vi "SQLite Count Template.vi"(6 "Range":T1, 7 "Filter":cluster{}, 8 "Error in":errorcluster, 10 "Filter Fields":string[](array[combo]), 11 "SQLite Connection in":refnum<class "Connection.lvclass">) -> (0 "Error out":errorcluster, 2 "Count":i32, 3 "SQLite Connection out":refnum<class "Connection.lvclass">)   [LabVIEW 2021]
uses:
  <vilib>/drjdpowell/SQLite Library/SQL Statement/SQL Statement.lvclass
  <vilib>/drjdpowell/SQLite Library/SQL Connection/Connection.lvclass
  edt.lib/sqlite.lib/EDT SQLite+.lvlib
  edt.lib/sqlite.lib/SQLite Range.ctl
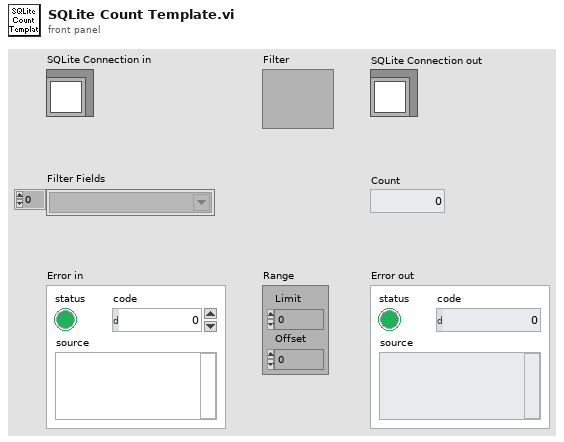
[diagram p1: front panel]
types:
  T1 = typedef "EDT SQLite+.lvlib/SQLite Range.ctl" = cluster{"Limit":i32, "Offset":i32}
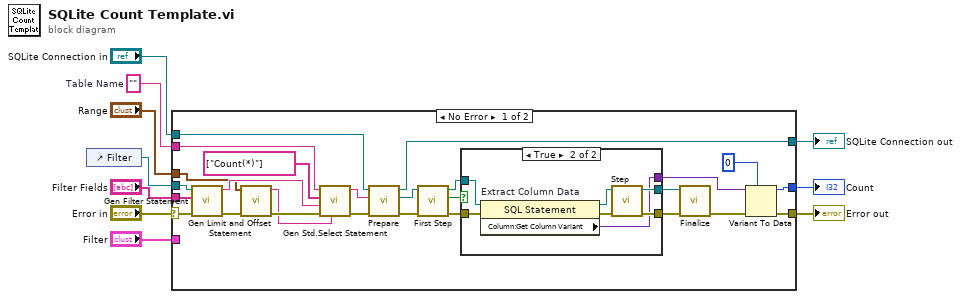
[diagram p0: block diagram]
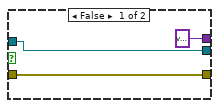
[diagram p2: hidden frame]
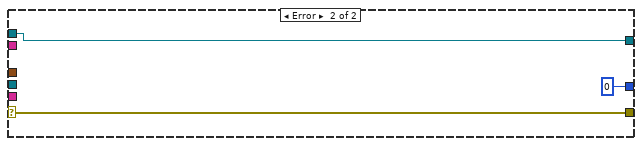
[diagram p3: hidden frame]
diagram:
  w5 = ""  # Table Name
  n1 = control-ref of="Filter"() -> (w4:refnum<vi>)
  n2 = case shown="No Error" "Error in" {
    selector: "Error in" -> [w24 w49]
    tunnel: [w12 w49] -> w9
    tunnel: "Filter" -> [_ _]
    tunnel: [w14 0] -> w1
    tunnel: "SQLite Connection in" -> [w22 w48]
    tunnel: [w21 w48] -> w6
    tunnel: w5 -> [w27 _]
    tunnel: w4 -> [w25 _]
    tunnel: "Filter Fields" -> [w26 _]
    tunnel: "Range" -> [w18 _]
    frame No Error {
      n3 = call "Gen Filter Statement.vi"("error in"=w24, "Columns"=w26, "Filter Cluster in"=w25) -> ("error out"=w20:errorcluster, "Filter String"=w23:string)  [unwired: 7 in]
      n4 = call "Gen Limit and Offset Statement.vi"("error in"=w20, "Range"=w18) -> ("error out"=w19:errorcluster, "Limit and Offset Statement"=w17:string)  [unwired: 8 in]
      n5 = call "Gen Std.Select Statement.vi"("Range String"=w17, "Error in"=w19, "Filter String"=w23, "Fields"=string[] ["Count(*)"], "Table Name"=w27) -> ("Error out"=w16:errorcluster, "String"=w28:string)  [unwired: 5 in]
      n6 = call <vilib>:"Prepare.vi"("error in (no error)"=w16, "SQL"=w28, "SQLite Connection in"=w22) -> ("error out"=w34:errorcluster, "SQL Statement"=w33:refnum<class "SQL Statement.lvclass">, "SQLite Connection"=w21:refnum<class "Connection.lvclass">)  [unwired: 4 in, 2 out]
      n7 = call <vilib>:"First Step.vi"("error in (no error)"=w34, "SQL Statement in"=w33) -> ("error out"=w31:errorcluster, "Row returned"=w30:bool, "SQL Statement"=w32:refnum<class "SQL Statement.lvclass">)  [unwired: 7 in]
      n8 = case "Results returned?" shown="True" w30 {
        tunnel: [w39 w46] -> w35
        tunnel: [w38 w45] -> w36
        tunnel: w32 -> [w39 w44]
        tunnel: w31 -> [w38 w43]
        tunnel: [variant ("Column:Get Column Variant") w42] -> w29
        frame False {
        }
        frame True {
          n9 = property on="Extract Column Data" class="SQL Statement"(reference=w44, error in=w43) -> (reference out=w41:refnum<class "SQL Statement.lvclass">, error out=w40:errorcluster, "Column:Get Column Variant"=w42:variant)
          n10 = call <vilib>:"Step.vi"("error in (no error)"=w40, "SQL Statement in"=w41) -> ("error out"=w45:errorcluster, "SQL Statement"=w46:refnum<class "SQL Statement.lvclass">)  [unwired: 7 in, 1 out]
        }
      }
      n11 = call <vilib>:"Finalize.vi"("error in (no error)"=w36, "SQL Statement in"=w35) -> ("error out"=w13:errorcluster)  [unwired: 9 in]
      n12 = Variant To Data(error in=w13, type=0, Variant=w29) -> (data=w14:i32, error out=w12:errorcluster)
    }
    frame Error {
    }
  }
  "Error out" <- w9
  "SQLite Connection out" <- w6
  "Count" <- w1
